vi "Bundle Script_Named (Un)Bundler Insert.vi"(6 "Dialog Choice":enum32{"Choice 1", "Choice 2"}(radio), 8 "error in":errorcluster, 10 "Selected Items (tags)":string[](array[string]), 11 "Affected Items":T1) -> (0 "error out":errorcluster, 2 "Objects":refnum<vi>[](array[refnum]))   [LabVIEW 2023]
uses:
  top/BundleMagic.ctl
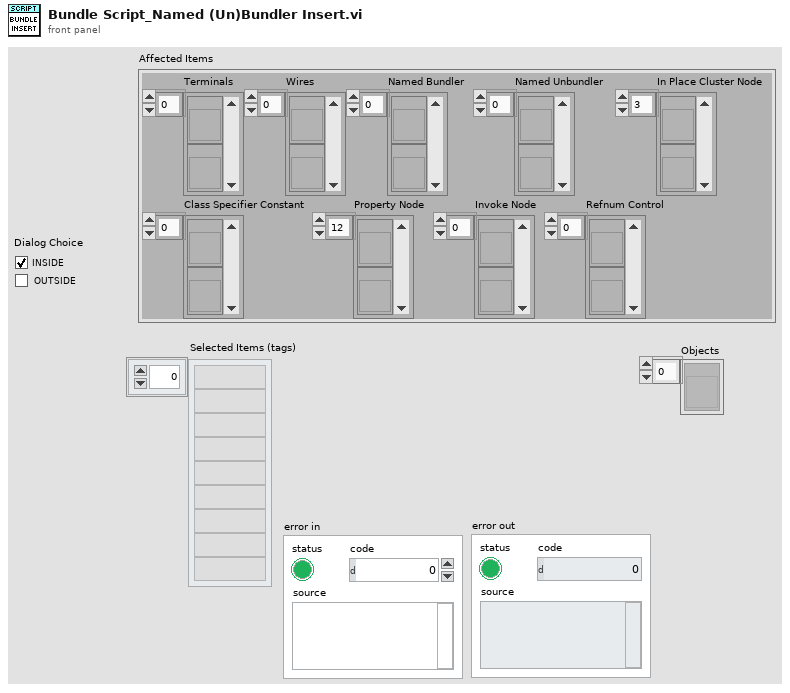
[diagram p1: front panel]
types:
  T1 = typedef "BundleMagic.ctl" = cluster{"Terminals":refnum<vi>[], "Wires":refnum<vi>[], "Named Bundler":refnum<vi>[], "Named Unbundler":refnum<vi>[], "In Place Cluster Node":refnum<vi>[], "Class Specifier Constant":refnum<vi>[], "Property Node":refnum<vi>[], "Invoke Node":refnum<vi>[], "Refnum Control":refnum<vi>[]}
  T2 = enum16{"Named Bundler", "Named Unbundler", "In Place", "None"}
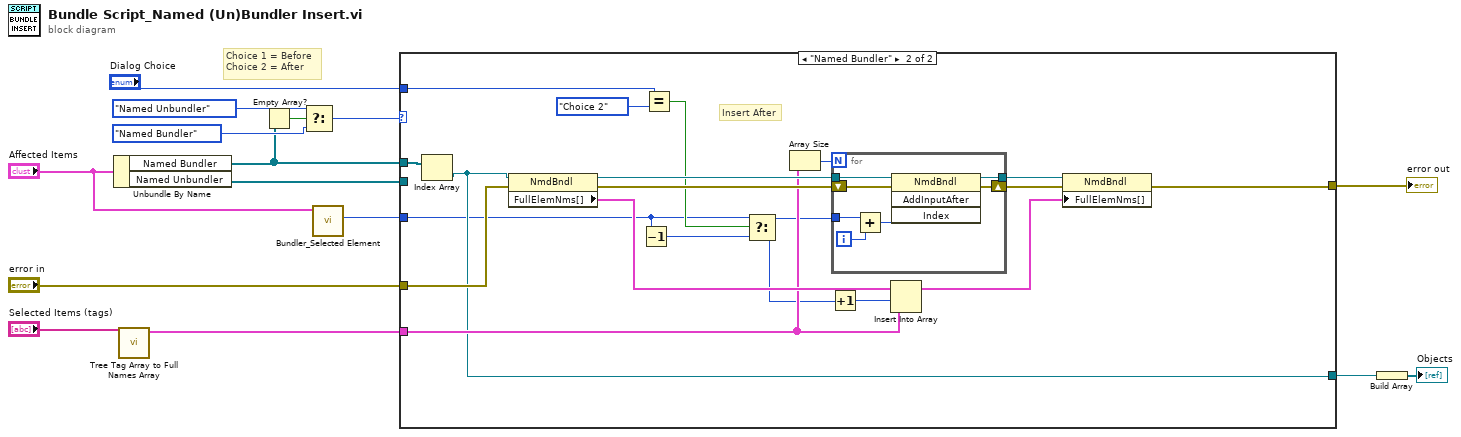
[diagram p0: block diagram]
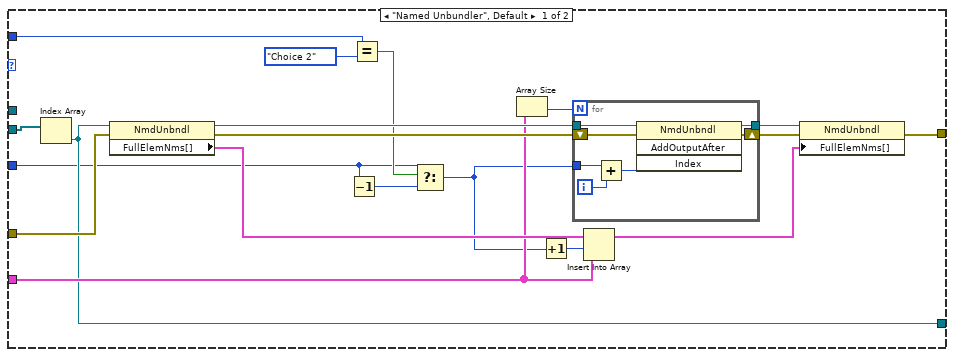
[diagram p2: hidden frame]
diagram:
  # "Choice 1 = Before\nChoice 2 = After"
  n1 = Unbundle By Name("Affected Items") -> ("Named Bundler"=w9:refnum<vi>[], "Named Unbundler"=w10:refnum<vi>[])
  n2 = call "Tree Tag Array to Full Names Array.vi"("Selected Items Tags"="Selected Items (tags)") -> ("Tree Item Values (nested form)"=w3:cluster{"Array":string[]}[])  [unwired: 6 in, 4 out]
  n3 = Empty Array?(array=w9) -> (empty?=w14:bool)
  n4 = Select(t=T2."Named Unbundler" ("Bundler Type"), s=w14, f=T2."Named Bundler" ("Bundler Type")) -> (s? t:f=w11:T2)
  n5 = call "Bundler_Selected Element.vi"("Affected Items"="Affected Items") -> ("index of element"=w1:i32)  [unwired: 5 in, 5 out]
  n6 = case shown="\"Named Bundler\"" w11 {
    tunnel: "error in" -> [w34 w60]
    tunnel: [w26 w52] -> w7
    tunnel: w3 -> [w28 w54]
    tunnel: "Dialog Choice" -> [w18 w44]
    tunnel: w10 -> [w25 _]
    tunnel: w9 -> [_ w51]
    tunnel: [w24 w50] -> w8
    tunnel: w1 -> [w16 w42]
    frame "Named Unbundler", Default {
      n7 = Index Array(array=w25) -> (element=w24:refnum<vi>)  [unwired: 1 in]
      n8 = property class="NmdUnbndl"(reference=w24, error in=w34) -> (reference out=w30:refnum<vi>, error out=w32:errorcluster, "FullElemNms[]"=w29:cluster{string[]}[])
      n9 = Decrement(x=w16) -> (x-1=w19:i32)
      n10 = Equal?(x=w18, y=enum32{"Choice 1", "Choice 2"}."Choice 2" ("Dialog Choice")) -> (x = y?=w20:bool)
      n11 = Select(t=w16, s=w20, f=w19) -> (s? t:f=w17:i32)
      n12 = Array Size(array=w28) -> (size(s)=w23:i32)
      n13 = Increment(x=w17) -> (x+1=w22:i32)
      n14 = for {
        N: w23 -> [_]
        shift-right: [w39] -> w31
        shift-left: w32 -> [w40]
        tunnel: w30 -> [w38]
        tunnel: [w41] -> w33
        tunnel: w17 -> [w36]
        i -> [w35]
        n15 = Add(x=w36, y=w35) -> (x+y=w37:i32)
        n16 = invoke class="NmdUnbndl" method="AddOutputAfter"(reference=w38, error in=w40, "Index"=w37) -> (reference out=w41:refnum<vi>, error out=w39:errorcluster)  [unwired: 1 in, 2 out]
      }
      n17 = Insert Into Array(array=w29, index=w22, new element=w28) -> (w27:cluster{string[]}[])
      n18 = property class="NmdUnbndl"(reference=w33, error in=w31, "FullElemNms[]"=w27) -> (error out=w26:errorcluster)  [unwired: 1 out]
    }
    frame "Named Bundler" {
      # "Insert After"
      n19 = Index Array(array=w51) -> (element=w50:refnum<vi>)  [unwired: 1 in]
      n20 = property class="NmdBndl"(reference=w50, error in=w60) -> (reference out=w56:refnum<vi>, error out=w58:errorcluster, "FullElemNms[]"=w55:cluster{string[]}[])
      n21 = Decrement(x=w42) -> (x-1=w46:i32)
      n22 = Equal?(x=w44, y=enum32{"Choice 1", "Choice 2"}."Choice 2" ("Dialog Choice")) -> (x = y?=w47:bool)
      n23 = Select(t=w42, s=w47, f=w46) -> (s? t:f=w43:i32)
      n24 = Array Size(array=w54) -> (size(s)=w49:i32)
      n25 = Increment(x=w43) -> (x+1=w48:i32)
      n26 = for {
        N: w49 -> [_]
        shift-right: [w65] -> w57
        shift-left: w58 -> [w66]
        tunnel: w56 -> [w64]
        tunnel: [w67] -> w59
        tunnel: w43 -> [w62]
        i -> [w61]
        n27 = Add(x=w62, y=w61) -> (x+y=w63:i32)
        n28 = invoke class="NmdBndl" method="AddInputAfter"(reference=w64, error in=w66, "Index"=w63) -> (reference out=w67:refnum<vi>, error out=w65:errorcluster)  [unwired: 1 in, 2 out]
      }
      n29 = Insert Into Array(array=w55, index=w48, new element=w54) -> (w53:cluster{string[]}[])
      n30 = property class="NmdBndl"(reference=w59, error in=w57, "FullElemNms[]"=w53) -> (error out=w52:errorcluster)  [unwired: 1 out]
    }
  }
  "error out" <- w7
  n31 = Build Array(w8) -> (→"Objects":refnum<vi>[])
